vi "UDP Data Link - Configuration Utilities - Initialize Device Sections and Channels.vi"(8 "error in (no error)":errorcluster, 11 "Item Ref out":T1 format="%.0x") -> (0 "error out":errorcluster, 3 "Parent Ref out":T1 format="%.0x")   [LabVIEW 2012, in "UDP Data Link System Explorer.lvlib"]
doc: "Add Status Channels and Receive (Rx) Channels Section to the system definition."
uses:
  UDP Data Link System Explorer.lvlib
  <vilib>/NI Veristand/Custom Device API/Custom Device Item Ref.ctl
  <vilib>/NI Veristand/Custom Device API/Custom Device Channel.ctl
  <vilib>/NI Veristand/Custom Device API/Custom Device Channel Type.ctl
  Shared/UDP Data Link Global.vi
  <vilib>/NI Veristand/Custom Device API/Custom Device API.lvlib
  Shared/UDP Data Link Shared.lvlib
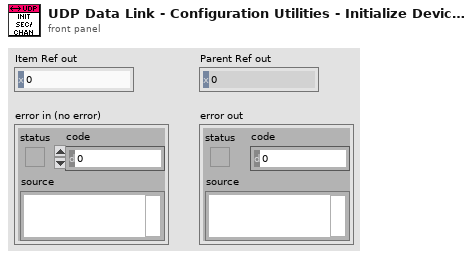
[diagram p1: front panel]
types:
  T1 = typedef "Custom Device API.lvlib/Custom Device Item Ref.ctl" = u64
  T2 = typedef "Custom Device API.lvlib/Custom Device Channel.ctl" = cluster{"Type":T3, "Units":string, "Default Value":dbl, "Faultable":bool, "Scalable":bool}
  T3 = typedef "Custom Device API.lvlib/Custom Device Channel Type.ctl" = enum16{"Input", "Output"}
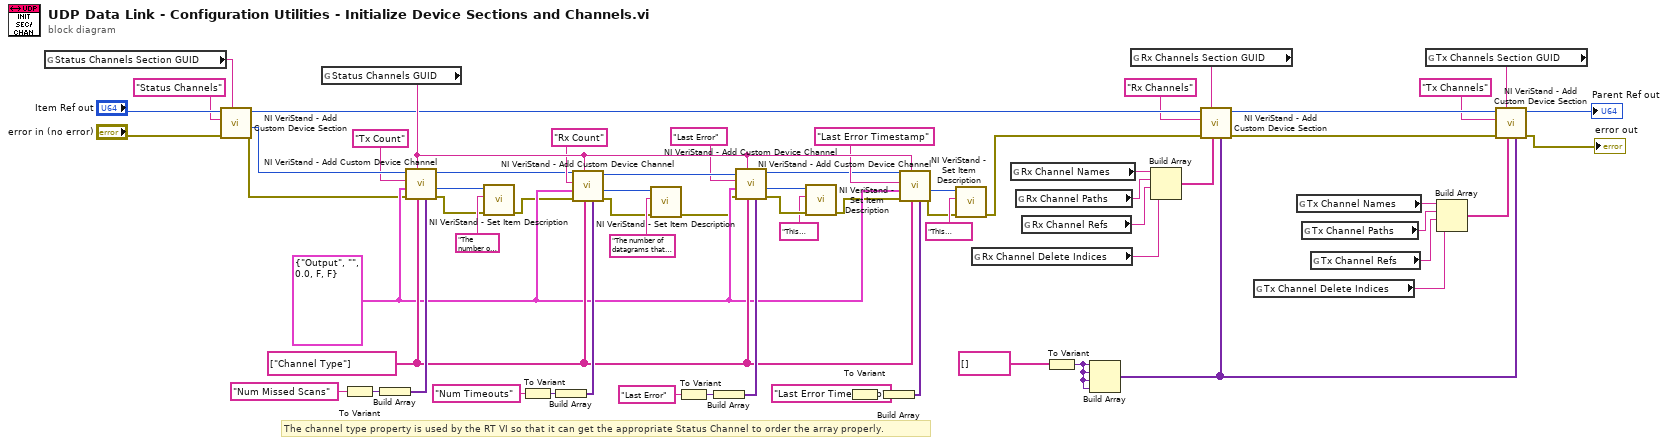
[diagram p0: block diagram]
diagram:
  w46 = string[] ["Channel Type"] ("Property names")
  w45 = T2 {"Type"=enum."Output", "Units"="", "Default Value"=0.0, "Faultable"=FALSE, "Scalable"=FALSE} ("Channel")
  # "The channel type property is used by the RT VI so that it can get the appropriate Status Channel to order the array properly."
  n1 = global read "UDP Data Link Global.vi" "Status Channels Section GUID"() -> (w64:string)
  n2 = call <vilib>:"NI VeriStand - Add Custom Device Section.vi"("GUID (Default Section)"=w64, "error in (no error)"="error in (no error)", "Section Name"="Status Channels", "Parent Ref in"="Item Ref out") -> ("error out"=w35:errorcluster, "Section Ptr"=w34:T1, "Parent Ref out"=w60:T1)  [unwired: 4 in, 1 out]
  n3 = global read "UDP Data Link Global.vi" "Status Channels GUID"() -> (w65:string)
  n4 = To Variant(anything="Num Missed Scans" ("String")) -> (Variant=w48:variant)
  n5 = Build Array(w48) -> (w49:variant[])
  n6 = call <vilib>:"NI VeriStand - Add Custom Device Channel.vi"("Property Values"=w49, "Property names"=w46, "GUID (Default Channel)"=w65, "error in (no error)"=w35, "Channel"=w45, "Channel Name"="Tx Count", "Parent Ref in"=w34) -> ("error out"=w32:errorcluster, "Channel Ref"=w33:T1, "Parent Ref out"=w39:T1)  [unwired: 1 in, 1 out]
  n7 = call <vilib>:"NI VeriStand - Set Item Description.vi"("error in (no error)"=w32, "Description"="The number of datagrams that have not been transmitted.", "Item Ref in"=w33) -> ("error out"=w41:errorcluster)  [unwired: 6 in, 2 out]
  n8 = To Variant(anything="Num Timeouts" ("String")) -> (Variant=w50:variant)
  n9 = Build Array(w50) -> (w52:variant[])
  n10 = call <vilib>:"NI VeriStand - Add Custom Device Channel.vi"("Property Values"=w52, "Property names"=w46, "GUID (Default Channel)"=w65, "error in (no error)"=w41, "Channel"=w45, "Channel Name"="Rx Count", "Parent Ref in"=w39) -> ("error out"=w38:errorcluster, "Channel Ref"=w37:T1, "Parent Ref out"=w40:T1)  [unwired: 1 in, 1 out]
  n11 = call <vilib>:"NI VeriStand - Set Item Description.vi"("error in (no error)"=w38, "Description"="The number of datagrams that have not been received.", "Item Ref in"=w37) -> ("error out"=w42:errorcluster)  [unwired: 6 in, 2 out]
  n12 = To Variant(anything="Last Error" ("String")) -> (Variant=w54:variant)
  n13 = Build Array(w54) -> (w55:variant[])
  n14 = call <vilib>:"NI VeriStand - Add Custom Device Channel.vi"("Property Values"=w55, "Property names"=w46, "GUID (Default Channel)"=w65, "error in (no error)"=w42, "Channel"=w45, "Channel Name"="Last Error", "Parent Ref in"=w40) -> ("error out"=w28:errorcluster, "Channel Ref"=w22:T1, "Parent Ref out"=w20:T1)  [unwired: 1 in, 1 out]
  n15 = call <vilib>:"NI VeriStand - Set Item Description.vi"("error in (no error)"=w28, "Description"="This Channel gives the last error of TCP Server. There is no distinction between error and warning.", "Item Ref in"=w22) -> ("error out"=w23:errorcluster)  [unwired: 6 in, 2 out]
  n16 = To Variant(anything="Last Error Timestamp" ("String")) -> (Variant=w56:variant)
  n17 = Build Array(w56) -> (w58:variant[])
  n18 = call <vilib>:"NI VeriStand - Add Custom Device Channel.vi"("Property Values"=w58, "Property names"=w46, "GUID (Default Channel)"=w65, "error in (no error)"=w23, "Channel"=w45, "Channel Name"="Last Error Timestamp", "Parent Ref in"=w20) -> ("error out"=w25:errorcluster, "Channel Ref"=w21:T1)  [unwired: 1 in, 2 out]
  n19 = call <vilib>:"NI VeriStand - Set Item Description.vi"("error in (no error)"=w25, "Description"="This Channel gives the System Time When the Channel \"Server Last Error\" was last updated.", "Item Ref in"=w21) -> ("error out"=w61:errorcluster)  [unwired: 6 in, 2 out]
  n20 = global read "UDP Data Link Global.vi" "Rx Channel Delete Indices"() -> (w4:string)
  n21 = global read "UDP Data Link Global.vi" "Rx Channel Names"() -> (w8:string)
  n22 = global read "UDP Data Link Global.vi" "Rx Channel Paths"() -> (w9:string)
  n23 = global read "UDP Data Link Global.vi" "Rx Channel Refs"() -> (w5:string)
  n24 = To Variant(anything=string[] []) -> (Variant=w1:variant)
  n25 = Build Array(w1, w1, w1, w1) -> (w6:variant[])
  n26 = global read "UDP Data Link Global.vi" "Rx Channels Section GUID"() -> (w66:string)
  n27 = Build Array(w8, w9, w5, w4) -> (w7:string[])
  n28 = call <vilib>:"NI VeriStand - Add Custom Device Section.vi"("Property Values"=w6, "Property names"=w7, "GUID (Default Section)"=w66, "error in (no error)"=w61, "Section Name"="Rx Channels", "Parent Ref in"=w60) -> ("error out"=w17:errorcluster, "Parent Ref out"=w18:T1)  [unwired: 2 in, 2 out]
  n29 = global read "UDP Data Link Global.vi" "Tx Channel Delete Indices"() -> (w2:string)
  n30 = global read "UDP Data Link Global.vi" "Tx Channel Names"() -> (w13:string)
  n31 = global read "UDP Data Link Global.vi" "Tx Channel Paths"() -> (w12:string)
  n32 = global read "UDP Data Link Global.vi" "Tx Channel Refs"() -> (w3:string)
  n33 = global read "UDP Data Link Global.vi" "Tx Channels Section GUID"() -> (w19:string)
  n34 = Build Array(w13, w12, w3, w2) -> (w11:string[])
  n35 = call <vilib>:"NI VeriStand - Add Custom Device Section.vi"("Property Values"=w6, "Property names"=w11, "GUID (Default Section)"=w19, "error in (no error)"=w17, "Section Name"="Tx Channels", "Parent Ref in"=w18) -> ("error out"=→"error out":errorcluster, "Parent Ref out"=→"Parent Ref out":T1)  [unwired: 2 in, 2 out]
